vi "Check Development data.vi"(3 "error in (no error)":errorcluster, 4 "Base Path":path=path "C:/ModisEdge/Scope/Test Sequence/Modis Edge Scope Test.seq", 5 "Sequence Context":refnum<k7>) -> (0 "error out":errorcluster, 2 "Report Text":string)   [LabVIEW 2015]
panel:
  out "file or folder exists?":bool
  out "Development Environment":string
  out "stripped path":path
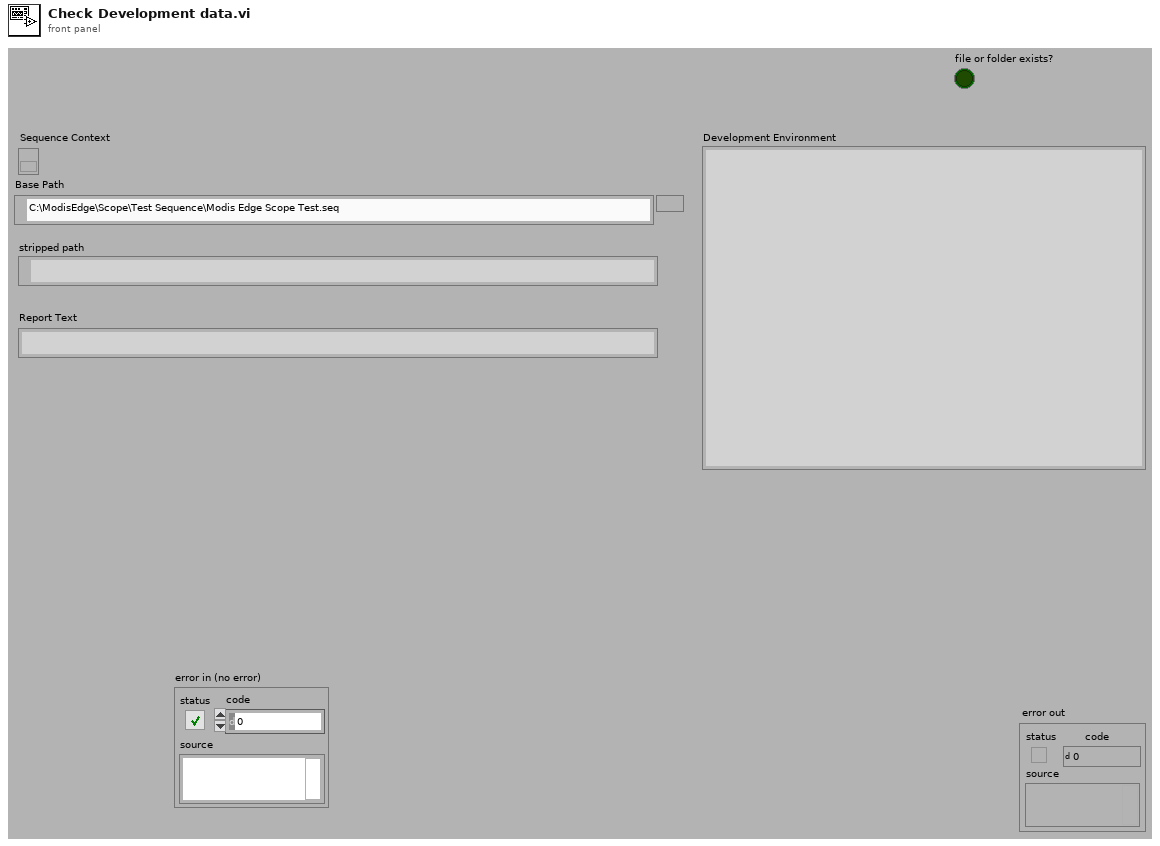
[diagram p1: front panel]
types:
  T1 = enum32{"invalid app kind", "Development System", "Run Time System", "Student Edition", "Embedded LabVIEW", "Evaluation", "Custom"}
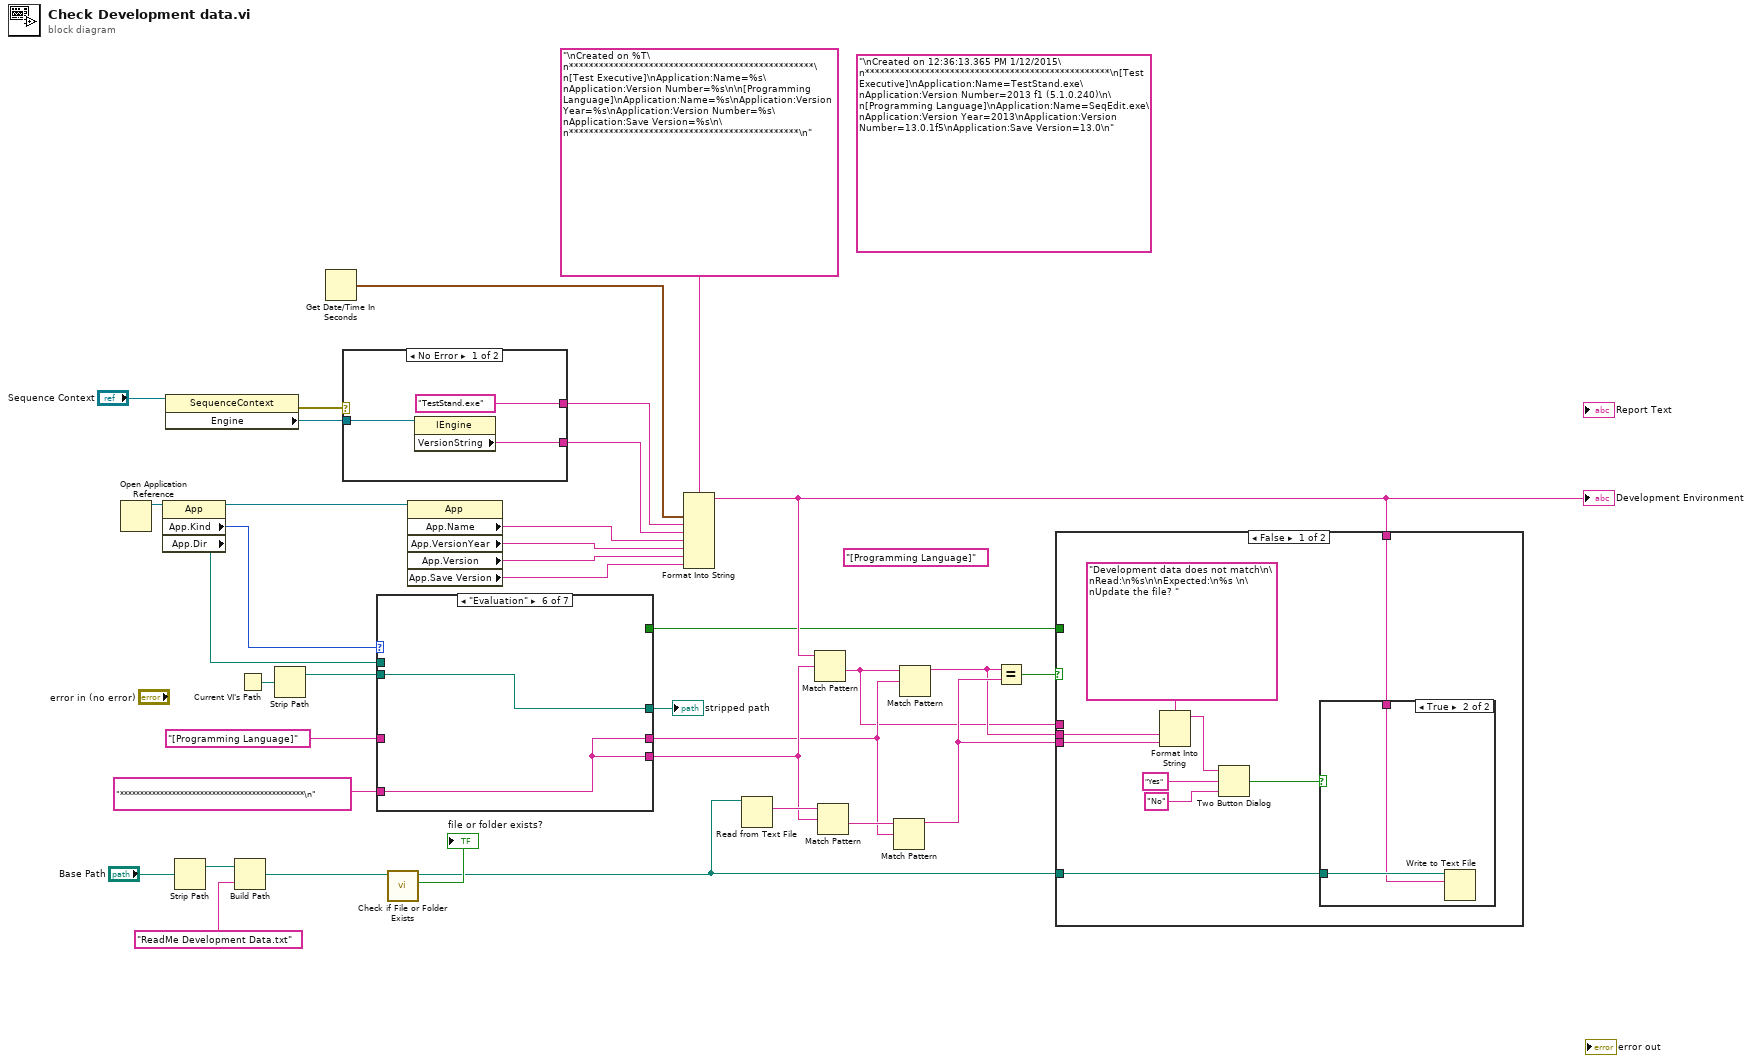
[diagram p0: block diagram]
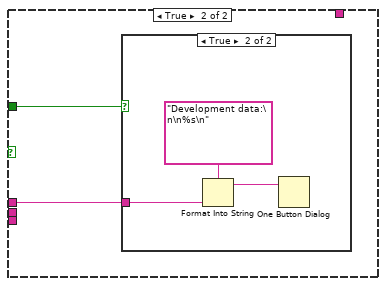
[diagram p3: hidden frame]
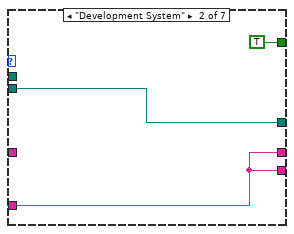
[diagram p7: hidden frame]
diagram:
  (unwired) "[Programming Language]"
  (unwired) "\nCreated on 12:36:13.365 PM 1/12/2015\n*************************************************\n[Test Executive]\nApplication:Name=TestStand.exe\nApplication:Version Number=2013 f1 (5.1.0.240)\n\n[Programming Language]\nApplication:Name=SeqEdit.exe\nApplication:Version Year=2013\nApplication:Version Number=13.0.1f5\nApplication:Save Version=13.0\n"
  n1 = Open Application Reference() -> (3:w30:refnum<vi>)  [unwired: 4 in, 1 out]
  n2 = property class="App"(reference=w30) -> (reference out=w29:refnum<vi>, "App.Kind"=w31:T1, "App.Dir"=w32:path)  [unwired: 1 in, 1 out]
  n3 = property class="SequenceContext"(reference="Sequence Context") -> (error out=w19:errorcluster, "Engine"=w23:refnum<k7>)  [unwired: 1 in, 1 out]
  n4 = Strip Path(path="Base Path") -> (stripped path=w16:path)  [unwired: 1 out]
  n5 = Build Path(base path=w16, name or relative path="ReadMe Development Data.txt") -> (appended path=w13:path)
  n6 = Current VI's Path() -> (path=w33:path)
  n7 = Strip Path(path=w33) -> (stripped path=w34:path)  [unwired: 1 out]
  n8 = Get Date/Time In Seconds() -> (seconds since 1Jan1904=w24:timestamp)
  n9 = case shown="No Error" w19 {
    tunnel: w23 -> [w38 _]
    tunnel: [w37 _] -> w20
    tunnel: ["TestStand.exe" _] -> w18
    frame No Error {
      n10 = property class="IEngine"(reference=w38) -> ("VersionString"=w37:string)  [unwired: 1 in, 2 out]
    }
    frame Error {
    }
  }
  n11 = case shown="\"Evaluation\"" w31 {
    tunnel: [w40 w43 w46 w48 w50 w52 w54] -> w35
    tunnel: w32 -> [_ _ w46 _ _ _ _]
    tunnel: w34 -> [w40 w43 _ w48 w50 w52 w54]
    tunnel: "**********************************************\n" -> [w39 w42 w44 w47 w49 w51 w53]
    tunnel: [w39 w42 w44 w47 w49 w51 w53] -> w5
    tunnel: [w39 w42 w45 w47 w49 w51 w53] -> w4
    tunnel: "[Programming Language]" -> [_ _ w45 _ _ _ _]
    tunnel: [_ TRUE _ _ _ _ _] -> w1
    frame "invalid app kind", Default {
    }
    frame "Development System" {
    }
    frame "Run Time System" {
    }
    frame "Student Edition" {
    }
    frame "Embedded LabVIEW" {
    }
    frame "Evaluation" {
    }
    frame "Custom" {
    }
  }
  "stripped path" <- w35
  n12 = call <vilib>:"Check if File or Folder Exists.vi"("path"=w13) -> ("file or folder exists?"=→"file or folder exists?":bool)  [unwired: 8 in, 2 out]
  n13 = property class="App"(reference=w29) -> ("App.Name"=w21:string, "App.VersionYear"=w27:string, "App.Version"=w26:string, "App.Save Version"=w25:string)  [unwired: 1 in, 2 out]
  n14 = Format Into String(format string="\nCreated on %T\n*************************************************\n[Test Executive]\nApplication:Name=%s\nApplication:Version Number=%s\n\n[Programming Language]\nApplication:Name=%s\nApplication:Version Year=%s\nApplication:Version Number=%s\nApplication:Save Version=%s\n\n**********************************************\n", w24, w18, w20, w21, w27, w26, w25) -> (resulting string=w12:string)  [unwired: 2 in, 1 out]
  "Development Environment" <- w12
  n15 = Read from Text File(file (use dialog)=w13) -> (text=w11:string)  [unwired: 3 in, 3 out]
  n16 = Match Pattern(string=w12, regular expression=w5) -> (after substring=w2:string)  [unwired: 1 in, 3 out]
  n17 = Match Pattern(string=w11, regular expression=w5) -> (after substring=w9:string)  [unwired: 1 in, 3 out]
  n18 = Match Pattern(string=w9, regular expression=w4) -> (before substring=w8:string)  [unwired: 1 in, 3 out]
  n19 = Match Pattern(string=w2, regular expression=w4) -> (before substring=w7:string)  [unwired: 1 in, 3 out]
  n20 = Equal?(x=w7, y=w8) -> (x = y?=w10:bool)
  n21 = case shown="False" w10 {
    tunnel: w13 -> [w63 _]
    tunnel: w12 -> [w62 _]
    tunnel: w8 -> [w56 _]
    tunnel: w7 -> [w55 _]
    tunnel: w2 -> [_ w67]
    tunnel: w1 -> [_ w66]
    frame False {
      n22 = Format Into String(format string="Development data does not match\n\nRead:\n%s\n\nExpected:\n%s \n\nUpdate the file? " ("message"), w55, w56) -> (resulting string=w58:string)  [unwired: 2 in, 1 out]
      n23 = Two Button Dialog(message=w58, 1:"No" ("F button name (\"Cancel\")"), 2:"Yes" ("T button name (\"OK\")")) -> (T button?=w61:bool)
      n24 = case shown="True" w61 {
        tunnel: w63 -> [_ w65]
        tunnel: w62 -> [_ w64]
        frame False {
        }
        frame True {
          n25 = Write to Text File(file (use dialog)=w65, text=w64) -> ()  [unwired: 2 in, 3 out]
        }
      }
    }
    frame True {
      n26 = case shown="True" w66 {
        tunnel: w67 -> [_ w68]
        frame False {
        }
        frame True {
          n27 = Format Into String(format string="Development data:\n\n%s\n" ("message"), w68) -> (resulting string=w69:string)  [unwired: 2 in, 1 out]
          n28 = One Button Dialog(message=w69) -> ()  [unwired: 1 in, 1 out]
        }
      }
    }
  }
